vi "theta to AX-Pos.vi"(4 "theta4a":dbl, 5 "theta3a":dbl, 6 "theta2a":dbl, 7 "theta1a":dbl) -> (0 "DEG 4":dbl, 1 "DEG 3":dbl, 2 "DEG 2":dbl, 3 "DEG1":dbl)   [LabVIEW 2017]
doc: "This VI Converts joint angle, theta, in dynamic equations to AX-12 servo angle, DEG."
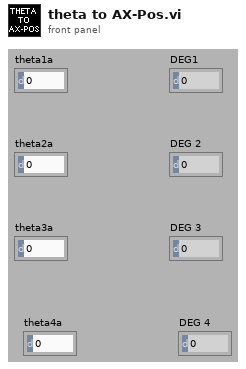
[diagram p1: front panel]
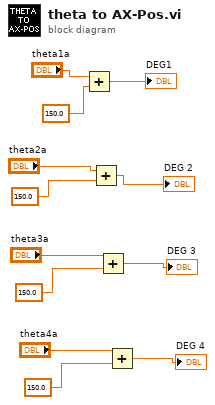
[diagram p0: block diagram]
diagram:
  n1 = Add(x="theta1a", y=150.0) -> (x+y=→"DEG1":dbl)
  n2 = Add(x="theta2a", y=150.0) -> (x+y=→"DEG 2":dbl)
  n3 = Add(x="theta3a", y=150.0) -> (x+y=→"DEG 3":dbl)
  n4 = Add(x="theta4a", y=150.0) -> (x+y=→"DEG 4":dbl)
